vi "Read Slew Rates.vi"(8 "Error In":errorcluster, 11 "Path":path) -> (0 "Error Out":errorcluster, 3 "Data Out":dbl[](array[numeric]))   [LabVIEW 2013]
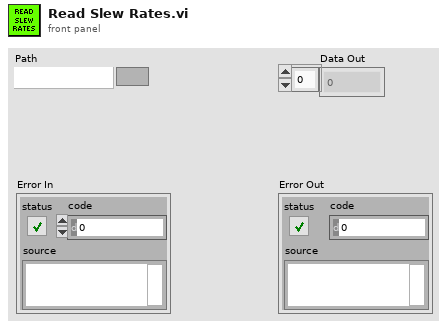
[diagram p1: front panel]
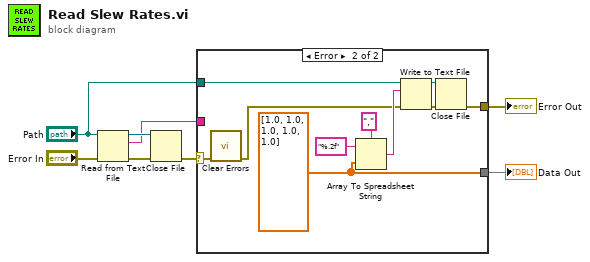
[diagram p0: block diagram]
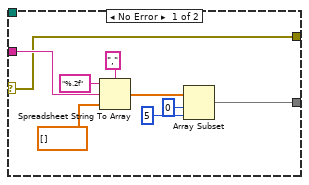
[diagram p2: hidden frame]
diagram:
  n1 = Read from Text File(file (use dialog)="Path", error in="Error In") -> (refnum out=w6:refnum<file>, text=w4:string, error out=w7:errorcluster)  [unwired: 2 in, 1 out]
  n2 = Close File(refnum=w6, error in=w7) -> (error out=w5:errorcluster)  [unwired: 1 out]
  n3 = case shown="Error" w5 {
    selector: w5 -> [w10 w27]
    tunnel: w4 -> [w15 _]
    tunnel: "Path" -> [_ w18]
    tunnel: [w10 w22] -> w2
    tunnel: [w9 w20] -> w1
    frame No Error {
      n4 = Spreadsheet String To Array(delimiter (Tab)=",", format string="%.2f", spreadsheet string=w15, array type (2D Dbl)=dbl[] []) -> (array=w11:dbl[])
      n5 = Array Subset(array=w11, index=0, length=5) -> (w9:dbl[])
    }
    frame Error {
      w20 = dbl[] [1.0, 1.0, 1.0, 1.0, 1.0]
      n6 = call <vilib>:"Clear Errors.vi"("error in (no error)"=w27) -> ("error out"=w19:errorcluster)  [unwired: 6 in]
      n7 = Array To Spreadsheet String(delimiter (Tab)=",", array=w20, 3:"%.2f" ("format string")) -> (spreadsheet string=w24:string)
      n8 = Write to Text File(file (use dialog)=w18, text=w24, error in=w19) -> (refnum out=w26:refnum<file>, error out=w25:errorcluster)  [unwired: 1 in, 1 out]
      n9 = Close File(refnum=w26, error in=w25) -> (error out=w22:errorcluster)  [unwired: 1 out]
    }
  }
  "Error Out" <- w2
  "Data Out" <- w1
